vi "Determine Warning Bad One.vi"(6 "최대":dbl, 7 "풍속":dbl, 8 "에러 입력(에러 없음)":cluster{"상태":bool, "코드":i32, "소스":string}, 9 "최저":dbl, 10 "최고":dbl, 11 "온도":dbl) -> (0 "에러 출력":cluster{"상태":bool, "코드":i32, "소스":string}, 1 "정지":bool, 2 "텍스트":string)   [LabVIEW 2010]
doc: "이것은 LabVIEW Core II에서 사용하는 연습문제 VI입니다. 향상될 필요가 있는 상속받은 코드의 예를 보여줍니다. 기능상의 변경없이 VI를 읽기 쉽고 유지하기 쉽게 개선하십시오."
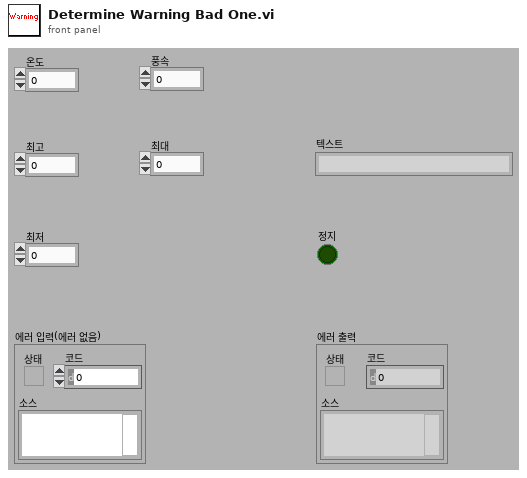
[diagram p1: front panel]
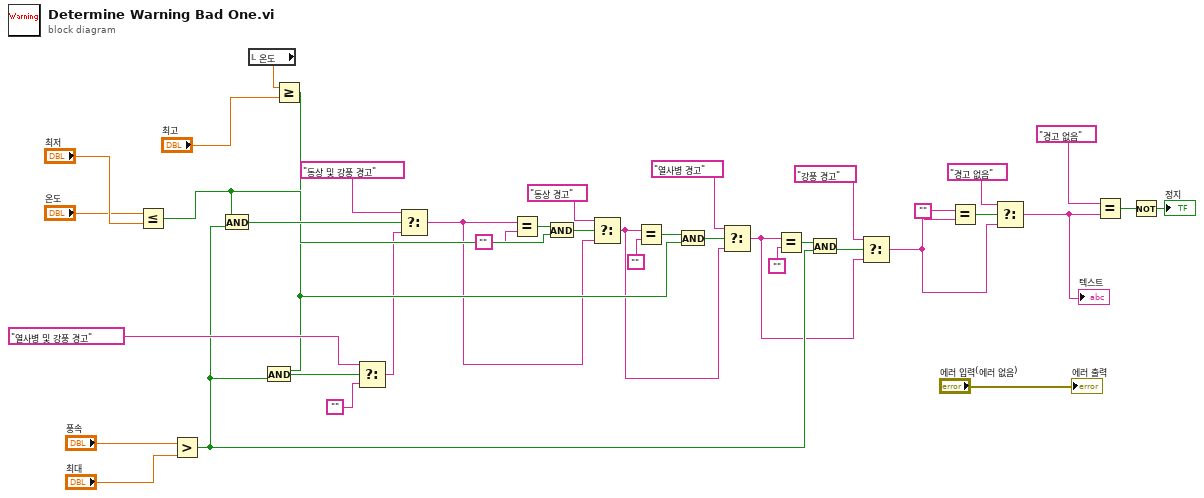
[diagram p0: block diagram]
diagram:
  n1 = Less Or Equal?(x="온도", y="최저") -> (x <= y?=w27:bool)
  n2 = Greater?(x="풍속", y="최대") -> (0:w21:bool)
  n3 = And(x=w27, y=w21) -> (x .and. y?=w29:bool)
  n4 = local read "온도"() -> (w8:dbl)
  n5 = Greater Or Equal?(x=w8, y="최고") -> (x >= y?=w22:bool)
  n6 = And(x=w22, y=w21) -> (x .and. y?=w32:bool)
  n7 = Select(t="열사병 및 강풍 경고", s=w32, f="") -> (s? t:f=w15:string)
  n8 = Select(t="동상 및 강풍 경고", s=w29, f=w15) -> (s? t:f=w14:string)
  n9 = Equal?(x=w14, y="") -> (x = y?=w28:bool)
  n10 = And(x=w28, y=w27) -> (x .and. y?=w26:bool)
  n11 = Select(t="동상 경고", s=w26, f=w14) -> (s? t:f=w12:string)
  n12 = Equal?(x=w12, y="") -> (x = y?=w24:bool)
  n13 = And(x=w24, y=w22) -> (x .and. y?=w25:bool)
  n14 = Select(t="열사병 경고", s=w25, f=w12) -> (s? t:f=w13:string)
  n15 = Equal?(x=w13, y="") -> (x = y?=w20:bool)
  n16 = And(x=w20, y=w21) -> (x .and. y?=w19:bool)
  n17 = Select(t="강풍 경고", s=w19, f=w13) -> (s? t:f=w10:string)
  n18 = Equal?(x=w10, y="") -> (x = y?=w16:bool)
  n19 = Select(t="경고 없음" ("f"), s=w16, f=w10) -> (s? t:f=w38:string)
  "텍스트" <- w38
  n20 = Equal?(x="경고 없음" ("f"), y=w38) -> (x = y?=w3:bool)
  n21 = Not(x=w3) -> (.not. x?=→"정지":bool)
  "에러 출력" <- "에러 입력(에러 없음)"
